vi "周期设置对话框.vi"() -> (2 "确定":bool, 3 "输出簇":T1)   [LabVIEW 2016]
uses:
  <vilib>/Utility/config.llb/Read Key (I32).vi
  <vilib>/Utility/config.llb/Read Key (Boolean).vi
  <vilib>/Utility/config.llb/Write Key (I32).vi
  <vilib>/Utility/config.llb/Write Key (Boolean).vi
  <vilib>/Utility/config.llb/NI_LVConfig.lvlib
panel:
  in  "总磷总氮":bool
  in  "氨氮":bool
  in  "CODCr":bool
  in  "多参数":bool
  in  "运行模式":enum16{"维护模式", "常规模式", "应急模式", "质控模式"}(ring)
  in  "运行间隔":i16=4 min=1 max=24
  in  "取消":bool
  in  "确定":bool
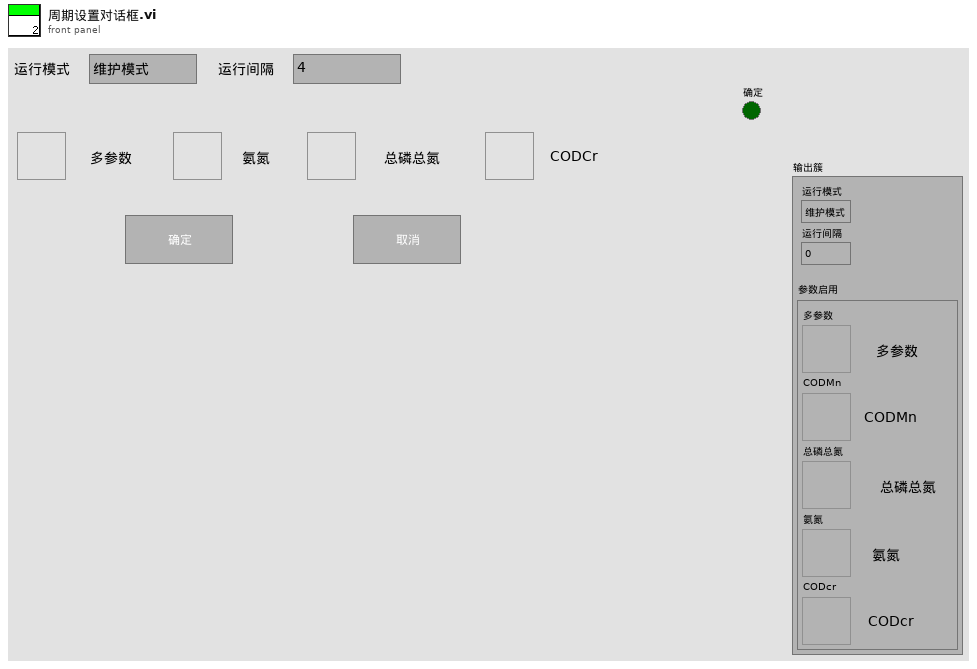
[diagram p1: front panel]
types:
  T1 = cluster{"运行模式":enum16{"维护模式", "常规模式", "应急模式", "质控模式"}, "运行间隔":i16, "参数启用":cluster{"多参数":bool, "CODMn":bool, "总磷总氮":bool, "氨氮":bool, "CODcr":bool}}
  T2 = typedef "NI_LVConfig.lvlib/Config Data RefNum.ctl" = refnum<k1>
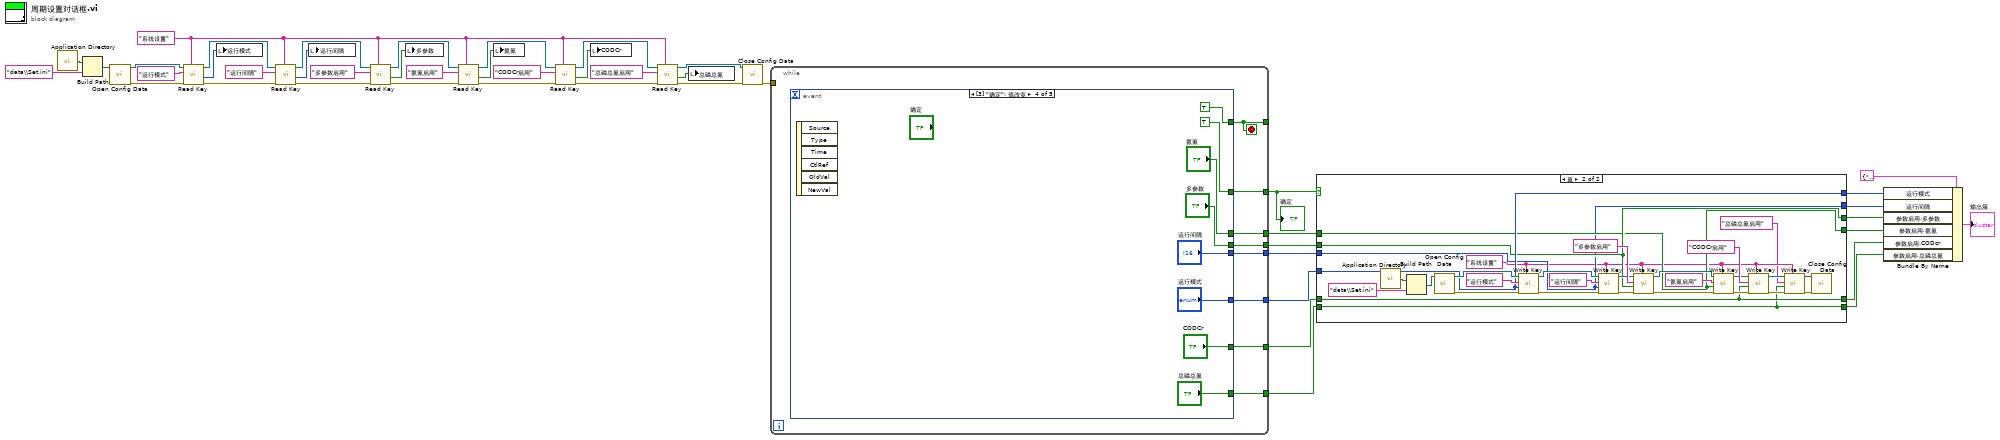
[diagram p0: block diagram]
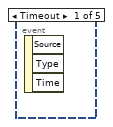
[diagram p3: hidden frame]
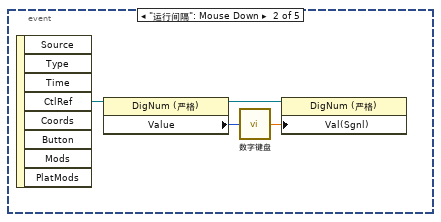
[diagram p4: hidden frame]
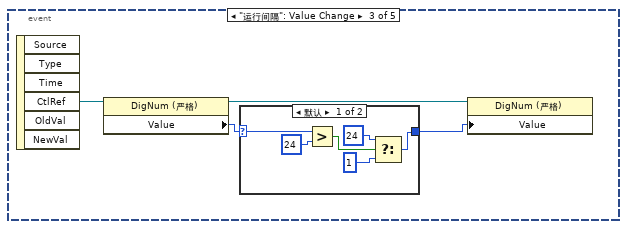
[diagram p5: hidden frame]
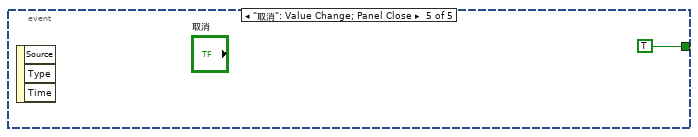
[diagram p7: hidden frame]
diagram:
  w3 = "系统设置" ("section")
  n1 = call <vilib>:"Application Directory.vi"() -> ("Application Directory"=w25:path)
  n2 = Build Path(base path=w25, name or relative path="data\\Set.ini" ("名称或相对路径")) -> (appended path=w27:path)
  n3 = call <vilib>:"Open Config Data.vi"("configuration file path"=w27) -> ("error out"=w24:errorcluster, "refnum"=w23:T2)  [unwired: 8 in, 1 out]
  n4 = call-poly <vilib>:"Read Key.vi"("section"=w3, "error in (no error)"=w24, "key"="运行模式" ("section"), "refnum"=w23) -> ("error out"=w29:errorcluster, "value"=w22:i32, "refnum out"=w28:T2)  [unwired: 4 in, 1 out]
  n5 = local write "运行模式"(w22) -> ()
  n6 = call-poly <vilib>:"Read Key.vi"("section"=w3, "error in (no error)"=w29, "key"="运行间隔" ("section"), "refnum"=w28) -> ("error out"=w36:errorcluster, "value"=w21:i32, "refnum out"=w34:T2)  [unwired: 4 in, 1 out]
  n7 = local write "运行间隔"(w21) -> ()
  n8 = call-poly <vilib>:"Read Key.vi"("section"=w3, "error in (no error)"=w36, "key"="多参数启用" ("section"), "refnum"=w34) -> ("error out"=w32:errorcluster, "value"=w20:bool, "refnum out"=w33:T2)  [unwired: 4 in, 1 out]
  n9 = local write "多参数"(w20) -> ()
  n10 = call-poly <vilib>:"Read Key.vi"("section"=w3, "error in (no error)"=w32, "key"="氨氮启用" ("section"), "refnum"=w33) -> ("error out"=w37:errorcluster, "value"=w19:bool, "refnum out"=w35:T2)  [unwired: 4 in, 1 out]
  n11 = local write "氨氮"(w19) -> ()
  n12 = call-poly <vilib>:"Read Key.vi"("section"=w3, "error in (no error)"=w37, "key"="CODCr启用" ("section"), "refnum"=w35) -> ("error out"=w5:errorcluster, "value"=w18:bool, "refnum out"=w7:T2)  [unwired: 4 in, 1 out]
  n13 = local write "CODCr"(w18) -> ()
  n14 = call-poly <vilib>:"Read Key.vi"("section"=w3, "error in (no error)"=w5, "key"="总磷总氮启用" ("section"), "refnum"=w7) -> ("error out"=w4:errorcluster, "value"=w1:bool, "refnum out"=w6:T2)  [unwired: 4 in, 1 out]
  n15 = local write "总磷总氮"(w1) -> ()
  n16 = call <vilib>:"Close Config Data.vi"("error in (no error)"=w4, "refnum"=w6) -> ("error out"=w17:errorcluster)  [unwired: 8 in, 1 out]
  n17 = while {
    tunnel: [w54] -> _
    tunnel: [w53] -> w46
    tunnel: [w52] -> w43
    tunnel: [w51] -> w42
    tunnel: [w50] -> w41
    tunnel: [w49] -> w44
    tunnel: [w48] -> w45
    tunnel: w17 -> [_]
    tunnel: [w47] -> w9
    stop <- w54 stop-if-true
    n18 = event shown="[3] \"确定\": 值改变" {
      selector: _ -> [_ _ _ _ _]
      dyn-events: _ -> [_ _ _ _ _]
      timeout: _ -> [_ _ _ _ _]
      tunnel: [_ _ _ TRUE TRUE] -> w54
      tunnel: [_ _ _ TRUE _] -> w53
      tunnel: [_ _ _ "多参数" _] -> w52
      tunnel: [_ _ _ "氨氮" _] -> w51
      tunnel: [_ _ _ "CODCr" _] -> w50
      tunnel: [_ _ _ "运行模式" _] -> w49
      tunnel: [_ _ _ "运行间隔" _] -> w48
      tunnel: [_ _ _ "总磷总氮" _] -> w47
      event Timeout {
        n19 = event-data() -> ()  [unwired: 1 in, 3 out]
      }
      event "运行间隔": Mouse Down {
        n20 = event-data() -> ("CtlRef"=w55:refnum<vi>)  [unwired: 1 in, 7 out]
        n21 = property class="DigNum (严格)"(reference=w55) -> (reference out=w57:refnum<vi>, "Value"=w58:i16)  [unwired: 1 in, 1 out]
        n22 = call "数字键盘.vi"("OldNumber"=w58) -> ("NewNumber"=w56:sgl)
        n23 = property class="DigNum (严格)"(reference=w57, "Val(Sgnl)"=w56) -> ()  [unwired: 1 in, 2 out]
      }
      event "运行间隔": Value Change {
        n24 = event-data() -> ("CtlRef"=w62:refnum<vi>)  [unwired: 1 in, 5 out]
        n25 = property class="DigNum (严格)"(reference=w62) -> (reference out=w60:refnum<vi>, "Value"=w61:i16)  [unwired: 1 in, 1 out]
        n26 = case shown="默认" w61 {
          selector: w61 -> [w65 w69]
          tunnel: [w64 w69] -> w59
          frame Default {
            n27 = Greater?(x=w65, y=i16 24) -> (0:w67:bool)
            n28 = Select(t=i16 24 ("y"), s=w67, f=i16 1) -> (s? t:f=w64:i16)
          }
          frame 1..24 {
          }
        }
        n29 = property class="DigNum (严格)"(reference=w60, "Value"=w59) -> ()  [unwired: 1 in, 2 out]
      }
      event "确定": Value Change {
        n30 = event-data() -> ()  [unwired: 1 in, 6 out]
      }
      event "取消": Value Change; Panel Close {
        n31 = event-data() -> ()  [unwired: 1 in, 3 out]
      }
    }
  }
  "确定" <- w46
  n32 = case shown="真" w46 {
    tunnel: w45 -> [_ w86]
    tunnel: w44 -> [_ w90]
    tunnel: w43 -> [_ w89]
    tunnel: w42 -> [_ w88]
    tunnel: w41 -> [_ w87]
    tunnel: [_ w90] -> w14
    tunnel: [_ w86] -> w13
    tunnel: [_ w89] -> w12
    tunnel: [_ w88] -> w11
    tunnel: [_ w87] -> w10
    tunnel: w9 -> [_ w79]
    tunnel: [_ w79] -> w8
    frame False {
    }
    frame True {
      w83 = "系统设置" ("section")
      n33 = call <vilib>:"Application Directory.vi"() -> ("Application Directory"=w93:path)
      n34 = Build Path(base path=w93, name or relative path="data\\Set.ini" ("名称或相对路径")) -> (appended path=w95:path)
      n35 = call <vilib>:"Open Config Data.vi"("configuration file path"=w95) -> ("error out"=w92:errorcluster, "refnum"=w91:T2)  [unwired: 8 in, 1 out]
      n36 = call-poly <vilib>:"Write Key.vi"("section"=w83, "error in (no error)"=w92, "value"=w90, "key"="运行模式" ("section"), "refnum"=w91) -> ("error out"=w97:errorcluster, "refnum out"=w96:T2)  [unwired: 4 in, 1 out]
      n37 = call-poly <vilib>:"Write Key.vi"("section"=w83, "error in (no error)"=w97, "value"=w86, "key"="运行间隔" ("section"), "refnum"=w96) -> ("error out"=w104:errorcluster, "refnum out"=w102:T2)  [unwired: 4 in, 1 out]
      n38 = call-poly <vilib>:"Write Key.vi"("section"=w83, "error in (no error)"=w104, "value"=w89, "key"="多参数启用" ("section"), "refnum"=w102) -> ("error out"=w100:errorcluster, "refnum out"=w101:T2)  [unwired: 4 in, 1 out]
      n39 = call-poly <vilib>:"Write Key.vi"("section"=w83, "error in (no error)"=w100, "value"=w88, "key"="氨氮启用" ("section"), "refnum"=w101) -> ("error out"=w105:errorcluster, "refnum out"=w103:T2)  [unwired: 4 in, 1 out]
      n40 = call-poly <vilib>:"Write Key.vi"("section"=w83, "error in (no error)"=w105, "value"=w87, "key"="CODCr启用" ("section"), "refnum"=w103) -> ("error out"=w85:errorcluster, "refnum out"=w84:T2)  [unwired: 4 in, 1 out]
      n41 = call-poly <vilib>:"Write Key.vi"("section"=w83, "error in (no error)"=w85, "value"=w79, "key"="总磷总氮启用" ("section"), "refnum"=w84) -> ("error out"=w80:errorcluster, "refnum out"=w81:T2)  [unwired: 4 in, 1 out]
      n42 = call <vilib>:"Close Config Data.vi"("error in (no error)"=w80, "refnum"=w81) -> ()  [unwired: 8 in, 2 out]
    }
  }
  n43 = Bundle By Name(cluster=T1 {"运行模式"=enum."维护模式", "运行间隔"=0, "参数启用"={"多参数"=FALSE, "CODMn"=FALSE, "总磷总氮"=FALSE, "氨氮"=FALSE, "CODcr"=FALSE}} ("输出簇"), "运行模式"=w14, "运行间隔"=w13, "参数启用.多参数"=w12, "参数启用.氨氮"=w11, "参数启用.CODcr"=w10, "参数启用.总磷总氮"=w8) -> (→"输出簇":T1)
